vi "Close_core.vi"(8 "error in (no error)":errorcluster, 11 "ctlRef_Maps in":refnum<class "ctlRef_Maps.lvclass">) -> (0 "error out":errorcluster)   [LabVIEW 2020, in "CtlReferences.lvlib" / "ctlRef_Maps.lvclass"]
uses:
  ctlRef_Maps.lvclass
  CtlReferences/CtlReferences.lvclass
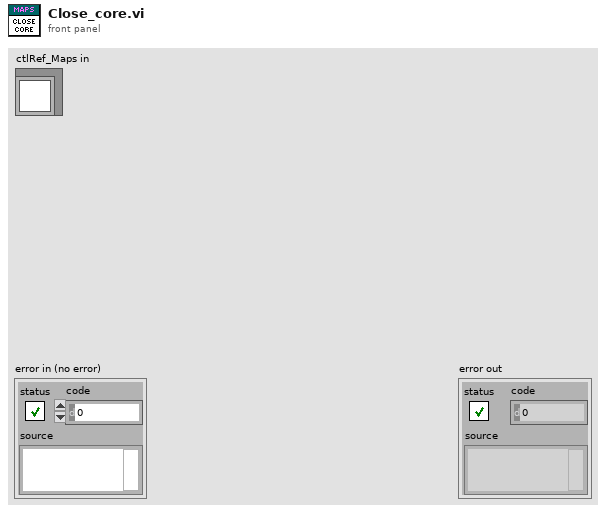
[diagram p1: front panel]
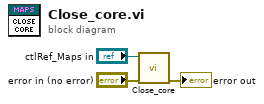
[diagram p0: block diagram]
diagram:
  n1 = call-parent "Close_core.vi"("error in (no error)"="error in (no error)", "CtlReferences in"="ctlRef_Maps in") -> ("error out"=→"error out":errorcluster)  [unwired: 9 in]
